vi "Filter Wheel Validate Move Command.vi"(7 "Filter Wheel in":refnum<class "Filter Wheel.lvclass">, 8 "error in (no error)":errorcluster, 10 "Filter Wheel Info":T2={"Num Wheels"=0, "Filters"=[], "Invalid Combinations"=[], "Addr"="", "Name"="", "Simulate"=FALSE, "Default Speed"=1000, "Homing"=[]} {"Default Speed" min=20 max=4000 step=10}, 11 "Move":T1) -> (0 "error out":errorcluster, 1 "already in pos?":bool, 2 "Valid?":bool, 3 "Move dup":T1)   [LabVIEW 2024]
uses:
  FW cmd Q Move Parameters.ctl
  Filter Wheel configuration.ctl
  Filter Wheel Object/Filter Wheel Details.ctl
  Filter Wheel Arduino Control/Filter Wheel Arduino Homing cluster.ctl
  Filter Wheel Object/Filter Wheel.lvclass
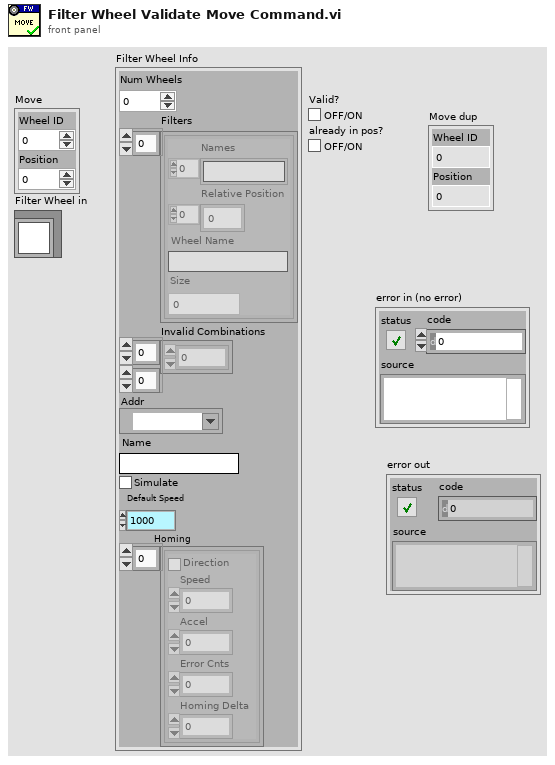
[diagram p1: front panel]
types:
  T1 = typedef "FW cmd Q Move Parameters.ctl" = cluster{"Wheel ID":i32, "Position":i32}
  T2 = typedef "Filter Wheel.lvclass/Filter Wheel configuration.ctl" = cluster{"Num Wheels":i32, "Filters":T3[], "Invalid Combinations":i32[][], "Addr":refnum<visa-resource-name>, "Name":string, "Simulate":bool, "Default Speed":u16, "Homing":T4[]}
  T3 = typedef "Filter Wheel.lvclass/Filter Wheel Details.ctl" = cluster{"Names":string[], "Relative Position":i32[], "Wheel Name":string, "Size":i32}
  T4 = typedef "Filter Wheel Arduino Homing cluster.ctl" = cluster{"Direction":bool, "Speed":i32, "Accel":i32, "Error Cnts":i32, "Homing Delta":i32}
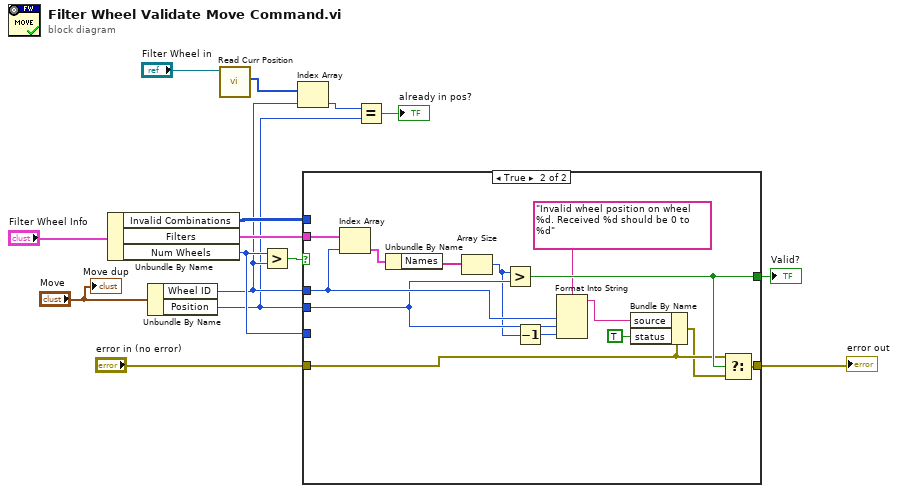
[diagram p0: block diagram]
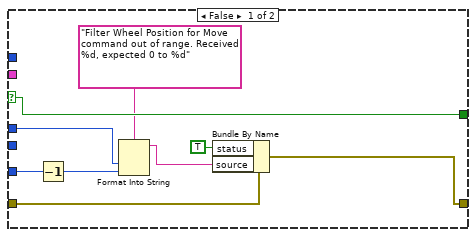
[diagram p2: hidden frame]
diagram:
  n1 = Unbundle By Name("Filter Wheel Info") -> ("Invalid Combinations"=w12:i32[][], "Filters"=w14:T3[], "Num Wheels"=w9:i32)
  n2 = Unbundle By Name("Move") -> ("Wheel ID"=w4:i32, "Position"=w2:i32)
  n3 = call-dynamic "Read Curr Position.vi"("Filter Wheel in"="Filter Wheel in") -> ("Curr Position"=w5:i32[])  [unwired: 8 in, 2 out]
  n4 = Greater?(x=w9, y=w4) -> (0:w13:bool)
  n5 = Index Array(array=w5, index=w4) -> (element=w3:i32)
  n6 = case shown="True" w13 {
    selector: w13 -> [w24 _]
    tunnel: w14 -> [_ w38]
    tunnel: w4 -> [w20 w29]
    tunnel: w12 -> [_ _]
    tunnel: w2 -> [_ w28]
    tunnel: [w24 w35] -> w11
    tunnel: "error in (no error)" -> [w23 w34]
    tunnel: w9 -> [w19 _]
    tunnel: [w17 w31] -> w8
    frame False {
      n7 = Decrement(x=w19) -> (x-1=w16:i32)
      n8 = Format Into String(format string="Filter Wheel Position for Move command out of range. Received %d, expected 0 to %d", w20, w16) -> (resulting string=w18:string)  [unwired: 2 in, 1 out]
      n9 = Bundle By Name(cluster=w23, "status"=TRUE, "source"=w18) -> (w17:errorcluster)
    }
    frame True {
      n10 = Index Array(array=w38, index=w29) -> (element=w37:T3)
      n11 = Unbundle By Name(w37) -> ("Names"=w36:string[])
      n12 = Array Size(array=w36) -> (size(s)=w27:i32)
      n13 = Greater?(x=w27, y=w28) -> (0:w35:bool)
      n14 = Decrement(x=w27) -> (x-1=w26:i32)
      n15 = Format Into String(format string="Invalid wheel position on wheel %d. Received %d should be 0 to %d", w29, w28, w26) -> (resulting string=w25:string)  [unwired: 2 in, 1 out]
      n16 = Bundle By Name(cluster=w34, "source"=w25, "status"=TRUE) -> (w32:errorcluster)
      n17 = Select(t=w34, s=w35, f=w32) -> (s? t:f=w31:errorcluster)
    }
  }
  "error out" <- w8
  "Valid?" <- w11
  n18 = Equal?(x=w3, y=w2) -> (x = y?=→"already in pos?":bool)
  "Move dup" <- "Move"
